vi "PopulaListaCanais.vi"(2 "DadosCanais":T1[](array[typedef])) -> (16 "Strings":string[][](array[string]))   [LabVIEW 2017]
uses:
  Typedefs/Tipo_DadosCanal.ctl
  Typedefs/Tipo_TipoSinalSimulado.ctl
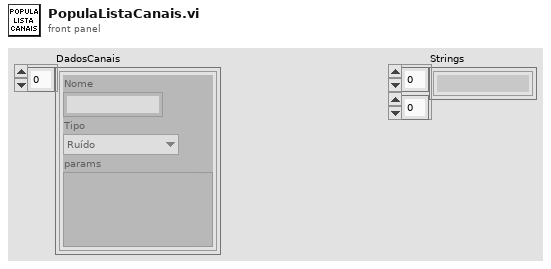
[diagram p1: front panel]
types:
  T1 = typedef "Tipo_DadosCanal.ctl" = cluster{"Nome":string, "Tipo":T2, "params":variant}
  T2 = typedef "Tipo_TipoSinalSimulado.ctl" = enum16{"Ruído", "Fasor", "Senóide", "Composto", "AM", "Proximidade", "Entreferro"}
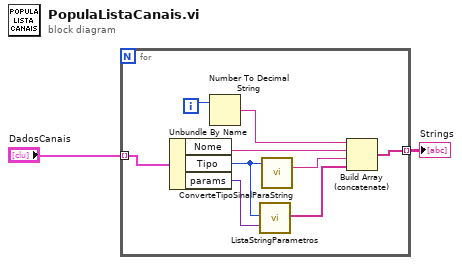
[diagram p0: block diagram]
diagram:
  n1 = for {
    tunnel: "DadosCanais" -> [w11] mode=indexing
    tunnel: [w6] -> w1 mode=indexing
    i -> [w10]
    n2 = Unbundle By Name(w11) -> ("Nome"=w8:string, "Tipo"=w5:T2, "params"=w4:variant)
    n3 = Number To Decimal String(number=w10) -> (decimal integer string=w9:string)  [unwired: 1 in]
    n4 = call "ListaStringParametros.vi"("Tipo"=w5, "Parametros"=w4) -> ("Parametros"=w3:string[])  [unwired: 17 in]
    n5 = call "ConverteTipoSinalParaString.vi"("Tipo"=w5) -> ("String"=w7:string)  [unwired: 18 in]
    n6 = Build Array (concatenate)(w9, w8, w7, w3) -> (w6:string[])
  }
  "Strings" <- w1
